vi "solar_app SOLARini Write (Section).vi"(6 "Comment (Create only)":string, 10 "Section":string) -> (2 "Found?":bool)   [LabVIEW 2018]
doc: "This writes a blank section to the solar.ini configuration file."
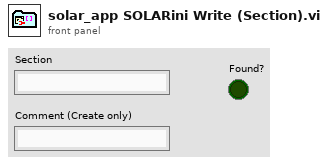
[diagram p1: front panel]
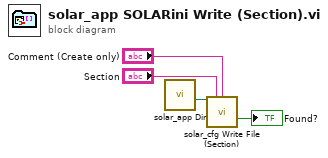
[diagram p0: block diagram]
diagram:
  n1 = call "solar_app Dir.vi"() -> ("solar.ini"=w4:path)  [unwired: 9 in, 2 out]
  n2 = call "solar_cfg Write File (Section).vi"("Config Path (*.ini)"=w4, "Section (\"\" = Use Filename)"="Section", "Comment"="Comment (Create only)") -> ("Found?"=→"Found?":bool)  [unwired: 10 in, 2 out]
